vi "Status Updated.vi"(8 "error in (no error)":errorcluster, 9 "Status":string, 10 "Name":string, 11 "Chat Window Model in":refnum<class "Chat Window Model.lvclass">) -> (0 "error out":errorcluster, 3 "Chat Window Model out":refnum<class "Chat Window Model.lvclass">)   [LabVIEW 2020, in "Chat Window Model.lvlib" / "Chat Window Model.lvclass"]
uses:
  Chat Window Model.lvclass
  C:/Program Files/National Instruments/LabVIEW 2020/vi.lib/ActorFramework/Actor/Actor.lvclass
  <vilib>/ActorFramework/Actor/Actor.lvclass/Actor.ctl
  Chat Window Model.lvclass/Chat Window Model.ctl
  Chat Window UI Controller/Chat Window UI Controller Messages/Update VI Title Msg/Update VI Title Msg.lvclass/Update VI Title Msg.ctl
  <vilib>/ActorFramework/Message Enqueuer/Message Enqueuer.lvclass/Message Enqueuer.ctl
  Msg Forward Interface Actor/Msg Forward Interface Actor Messages/Status Updated Msg/Status Updated Msg.lvclass/Status Updated Msg.ctl
  <vilib>/ActorFramework/Message Enqueuer/Enqueue.vi
  Chat Window UI Controller/Chat Window UI Controller Messages/Update VI Title Msg/Update VI Title Msg.lvclass
  C:/Program Files/National Instruments/LabVIEW 2020/vi.lib/ActorFramework/Message/Message.lvclass
  Msg Forward Interface Actor/Msg Forward Interface Actor Messages/Status Updated Msg/Status Updated Msg.lvclass
  <vilib>/ActorFramework/Message Priority Queue/Priority Enqueue.vi
  <vilib>/ActorFramework/Actor/Actor.lvclass
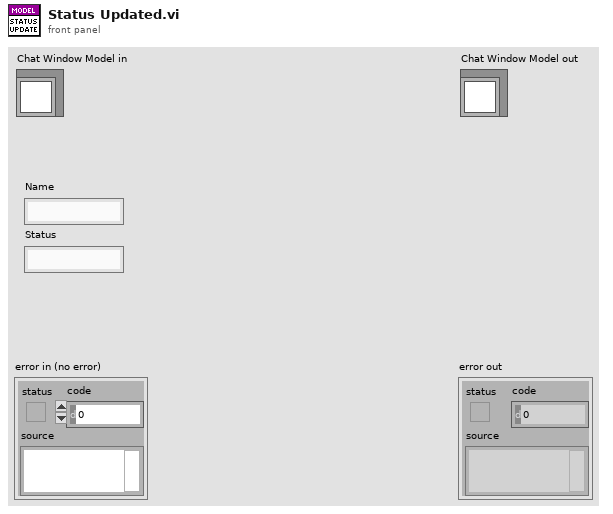
[diagram p1: front panel]
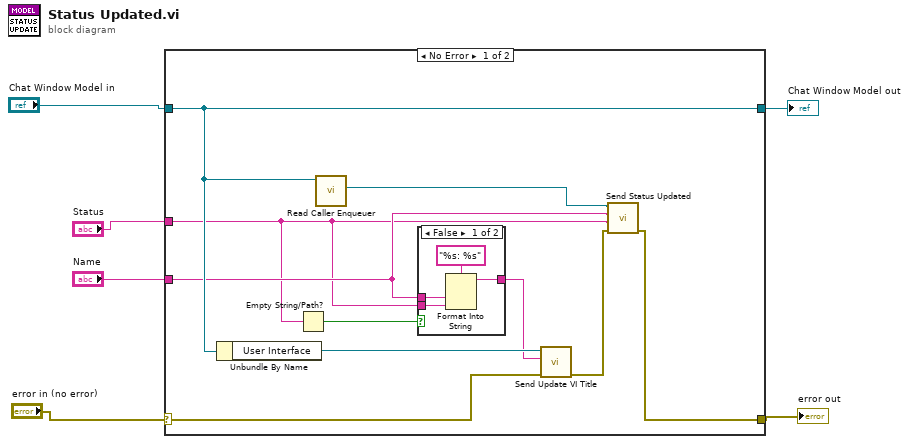
[diagram p0: block diagram]
diagram:
  n1 = case shown="No Error" "error in (no error)" {
    selector: "error in (no error)" -> [w14 w23]
    tunnel: [w7 w23] -> w4
    tunnel: [w16 w22] -> w6
    tunnel: "Chat Window Model in" -> [w16 w22]
    tunnel: "Status" -> [w9 _]
    tunnel: "Name" -> [w10 _]
    frame No Error {
      n2 = Unbundle By Name(w16) -> ("User Interface"=w15:refnum<class "Message Enqueuer.lvclass">)
      n3 = Empty String/Path?(string/path=w9) -> (empty?=w12:bool)
      n4 = call <vilib>:"Read Caller Enqueuer.vi"("Actor"=w16) -> ("Caller Enqueuer"=w11:refnum<class "Message Enqueuer.lvclass">)  [unwired: 10 in]
      n5 = case shown="False" w12 {
        tunnel: [w19 w21] -> w13
        tunnel: w10 -> [w18 w21]
        tunnel: w9 -> [w17 _]
        frame False {
          n6 = Format Into String(format string="%s: %s", w18, w17) -> (resulting string=w19:string)  [unwired: 2 in, 1 out]
        }
        frame True {
        }
      }
      n7 = call "Send Update VI Title.vi"("error in (no error)"=w14, "Window Title"=w13, "Message Enqueuer"=w15) -> ("error out"=w8:errorcluster)  [unwired: 7 in, 1 out]
      n8 = call "Send Status Updated.vi"("error in (no error)"=w8, "Status"=w9, "Name"=w10, "Message Enqueuer"=w11) -> ("error out"=w7:errorcluster)  [unwired: 6 in, 1 out]
    }
    frame Error {
    }
  }
  "error out" <- w4
  "Chat Window Model out" <- w6
